vi "test - Access priority for nested read.vi"(8 "error in (no error)":errorcluster, 11 "TestCase in":refnum<class "csm-ini-variable-addon.lvclass">) -> (0 "error out":errorcluster, 3 "TestCase out":refnum<class "csm-ini-variable-addon.lvclass">)   [LabVIEW 2017, in "csm-ini-variable-addon.lvclass"]
uses:
  csm-ini-variable-addon.lvclass
  51eeedc8-b31c-488c-8392-a86325f3fef9.vi
  d661d301-294d-4a40-9fe1-44519e1c8482.vi
  51eeedc8-b31c-488c-8392-a86325f3fef9.vi/de56416b-c5bf-46ee-94c0-236aa6ebb74d.vi
  d661d301-294d-4a40-9fe1-44519e1c8482.vi/5993f3dd-cba9-41f8-9723-db1d94748cc5.vi
  INI-Static-Variable-Support/_Support/global-csm-ini-db-change-flag.vi
  <vilib>/Utility/Data Type/Get Type Information.vi
  <userlib>/_NEVSTOP/Communicable State Machine(CSM)/addons/API-String-Arugments-Support/_Support/Data To SingleElementsArray_csm.vi
  INI-Static-Variable-Support/_Support/Parse Used Session and Name.vi
  <userlib>/_NEVSTOP/Communicable State Machine(CSM)/addons/API-String-Arugments-Support/_Support/Data To API String Arguments.vi
  INI-Static-Variable-Support/_Support/INI-FGV.vi
  INI-Static-Variable-Support/_Support/Populate String with INI Variable.vi
  <userlib>/_NEVSTOP/Communicable State Machine(CSM)/addons/API-String-Arugments-Support/_Support/Convert API String Arguments to Data(variant).vi
  <userlib>/_NEVSTOP/Communicable State Machine(CSM)/addons/API-String-Arugments-Support/_Support/SingleElementsArray To Data_csm.vi
  INI-Static-Variable-Support/INI-Static-Variable-Support.lvlib
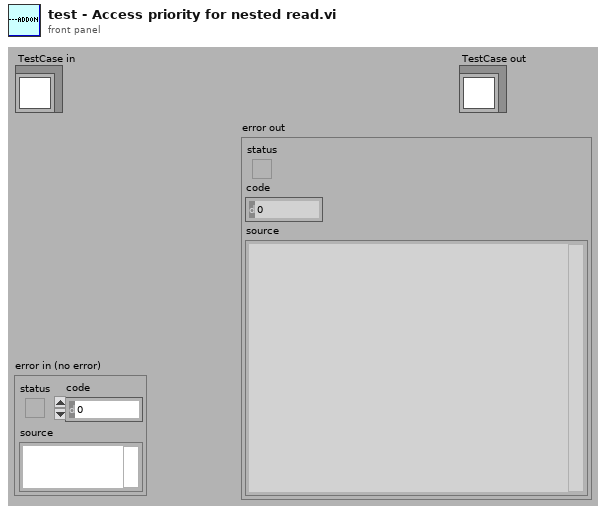
[diagram p1: front panel]
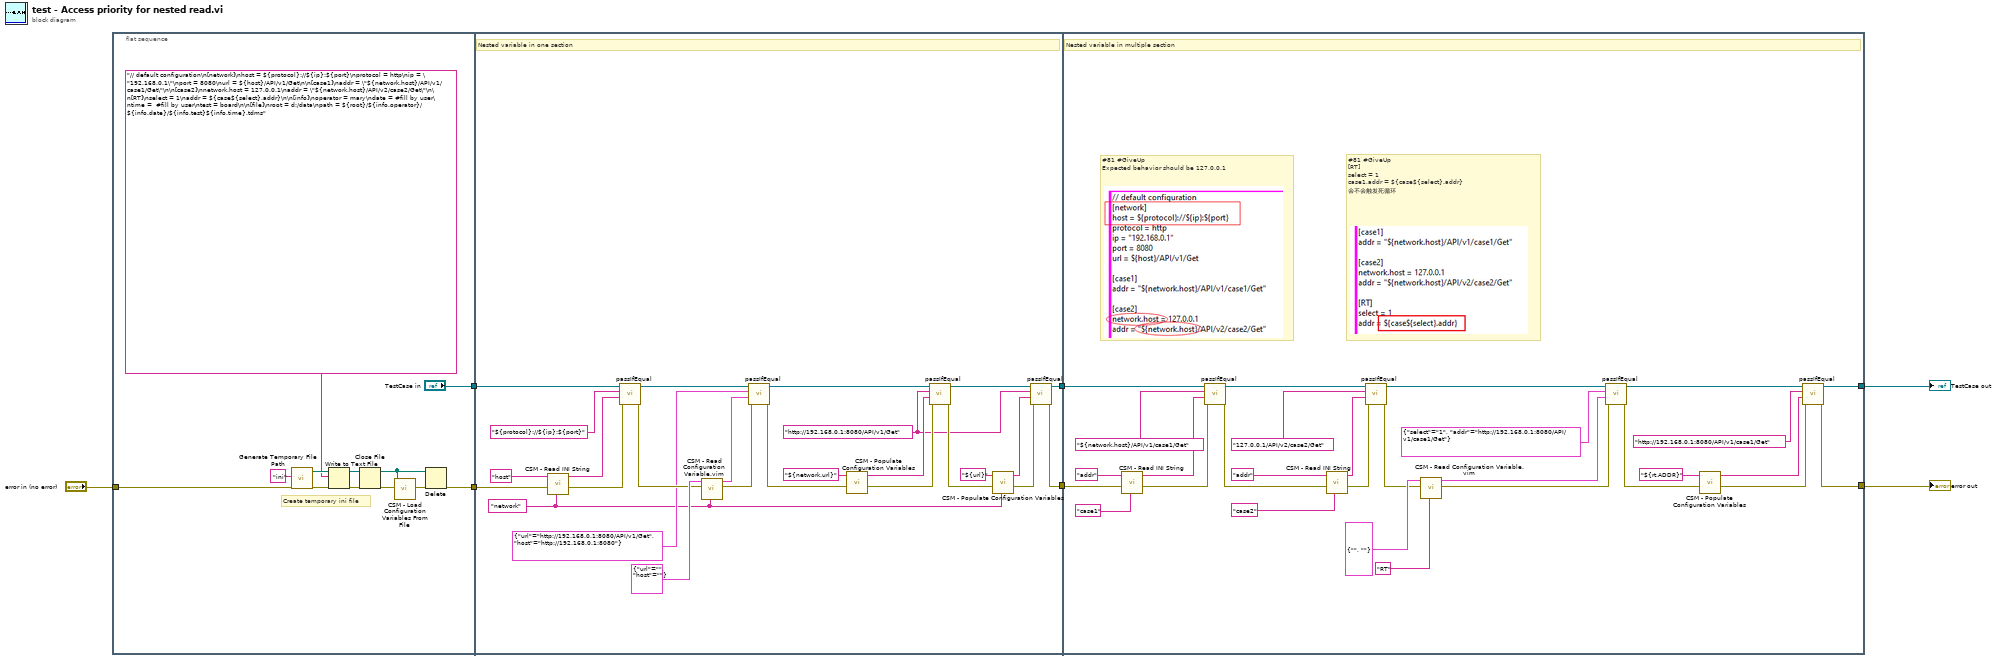
[diagram p0: block diagram]
diagram:
  n1 = flat-sequence {
    tunnel: "error in (no error)" -> [w10]
    tunnel: [w9] -> w6
    tunnel: ["TestCase in"] -> w5
    tunnel: w6 -> [w44]
    tunnel: w5 -> [w43]
    tunnel: [w21] -> w4
    tunnel: [w20] -> w3
    tunnel: w4 -> [w70]
    tunnel: w3 -> [w69]
    tunnel: [w47] -> w2
    tunnel: [w46] -> w1
    frame #0 {
      # "Create temporary ini file"
      n2 = call <vilib>:"Generate Temporary File Path.vi"("error in (no error)"=w10, "Temporary File Extension (tmp)"="ini") -> ("error out"=w19:errorcluster, "Unique Temporary File Path"=w16:path)  [unwired: 8 in]
      n3 = Write to Text File(file (use dialog)=w16, text="// default configuration\n[network]\nhost = ${protocol}://${ip}:${port}\nprotocol = http\nip = \"192.168.0.1\"\nport = 8080\nurl = ${host}/API/v1/Get\n\n[case1]\naddr = \"${network.host}/API/v1/case1/Get\"\n\n[case2]\nnetwork.host = 127.0.0.1\naddr = \"${network.host}/API/v2/case2/Get\"\n\n[RT]\nselect = 1\naddr = ${case${select}.addr}\n\n[info]\noperator = mary\ndate = #fill by user\ntime =  #fill by user\ntest = board\n\n[file]\nroot = d:/data\npath = ${root}/${info.operator}/${info.date}/${info.test}${info.time}.tdms", error in=w19) -> (refnum out=w15:refnum<file>, error out=w17:errorcluster)  [unwired: 1 in, 1 out]
      n4 = Close File(refnum=w15, error in=w17) -> (path=w11:path, error out=w14:errorcluster)
      n5 = call "CSM - Load Configuration Variables From File.vi"("error in (no error)"=w14, "Path"=w11) -> ("error out"=w12:errorcluster)  [unwired: 7 in]
      n6 = Delete(path (use dialog)=w11, error in=w12) -> (error out=w9:errorcluster)  [unwired: 3 in, 2 out]
    }
    frame #1 {
      w23 = "http://192.168.0.1:8080/API/v1/Get" ("${network.url}")
      w26 = "network" ("Section Name(\"\" as Default)")
      # "Nested variable in one section"
      n7 = call "CSM - Read INI String.vi"("Section Name(\"\" as Default)"=w26, "error in (no error)"=w44, "String in"="host") -> ("error out"=w41:errorcluster, "String out"=w42:string)  [unwired: 4 in, 1 out]
      n8 = call-dynamic "passIfEqual.vi"("error in (no error)"=w41, "y"=w42, "x"="${protocol}://${ip}:${port}" ("String in"), "TestCase in"=w43) -> ("error out"=w38:errorcluster, "TestCase out"=w36:refnum<class "csm-ini-variable-addon.lvclass">)  [unwired: 6 in]
      n9 = call "CSM - Read Configuration Variable.vim"("Section Name(\"\" as Default)"=w26, "error in (no error)"=w38, "config prototype(Cluster Prefered)"=cluster{"url":string, "host":string} {"url"="", "host"=""}) -> ("error out"=w37:errorcluster, "config out"=w35:cluster{"url":string, "host":string})  [unwired: 5 in]
      n10 = call-dynamic "passIfEqual.vi"("error in (no error)"=w37, "y"=w35, "x"=cluster{"url":string, "host":string} {"url"="http://192.168.0.1:8080/API/v1/Get", "host"="http://192.168.0.1:8080"} ("network.cluster"), "TestCase in"=w36) -> ("error out"=w31:errorcluster, "TestCase out"=w30:refnum<class "csm-ini-variable-addon.lvclass">)  [unwired: 6 in]
      n11 = call "CSM - Populate Configuration Variables.vi"("error in (no error)"=w31, "String in"="${network.url}") -> ("error out"=w28:errorcluster, "String out"=w29:string)  [unwired: 6 in]
      n12 = call-dynamic "passIfEqual.vi"("error in (no error)"=w28, "y"=w29, "x"=w23, "TestCase in"=w30) -> ("error out"=w27:errorcluster, "TestCase out"=w25:refnum<class "csm-ini-variable-addon.lvclass">)  [unwired: 6 in]
      n13 = call "CSM - Populate Configuration Variables.vi"("Section Name(\"\" as Default)"=w26, "error in (no error)"=w27, "String in"="${url}") -> ("error out"=w24:errorcluster, "String out"=w22:string)  [unwired: 5 in]
      n14 = call-dynamic "passIfEqual.vi"("error in (no error)"=w24, "y"=w22, "x"=w23, "TestCase in"=w25) -> ("error out"=w21:errorcluster, "TestCase out"=w20:refnum<class "csm-ini-variable-addon.lvclass">)  [unwired: 6 in]
    }
    frame #2 {
      # "#81 #GiveUp\nExpected behavior should be 127.0.0.1"
      # "Nested variable in multiple section"
      # "#81 #GiveUp\n[RT]\nselect = 1\ncase1.addr = ${case${select}.addr}\n会不会触发死循环"
      n15 = call "CSM - Read INI String.vi"("Section Name(\"\" as Default)"="case1" ("Section Name(\"\" as Default)"), "error in (no error)"=w70, "String in"="addr") -> ("error out"=w67:errorcluster, "String out"=w66:string)  [unwired: 4 in, 1 out]
      n16 = call-dynamic "passIfEqual.vi"("error in (no error)"=w67, "y"=w66, "x"="${network.host}/API/v1/case1/Get" ("case1.addr"), "TestCase in"=w69) -> ("error out"=w68:errorcluster, "TestCase out"=w65:refnum<class "csm-ini-variable-addon.lvclass">)  [unwired: 6 in]
      n17 = call "CSM - Read INI String.vi"("Section Name(\"\" as Default)"="case2" ("Section Name(\"\" as Default)"), "error in (no error)"=w68, "String in"="addr") -> ("error out"=w64:errorcluster, "String out"=w63:string)  [unwired: 4 in, 1 out]
      n18 = call-dynamic "passIfEqual.vi"("error in (no error)"=w64, "y"=w63, "x"="127.0.0.1/API/v2/case2/Get" ("case2.addr"), "TestCase in"=w65) -> ("error out"=w58:errorcluster, "TestCase out"=w57:refnum<class "csm-ini-variable-addon.lvclass">)  [unwired: 6 in]
      n19 = call "CSM - Read Configuration Variable.vim"("Section Name(\"\" as Default)"="RT" ("Section Name(\"\" as Default)"), "error in (no error)"=w58, "config prototype(Cluster Prefered)"=cluster{"select":string, "addr":string} {"select"="", "addr"=""}) -> ("error out"=w56:errorcluster, "config out"=w55:cluster{"select":string, "addr":string})  [unwired: 5 in]
      n20 = call-dynamic "passIfEqual.vi"("error in (no error)"=w56, "y"=w55, "x"=cluster{"select":string, "addr":string} {"select"="1", "addr"="http://192.168.0.1:8080/API/v1/case1/Get"} ("rt.cluster"), "TestCase in"=w57) -> ("error out"=w52:errorcluster, "TestCase out"=w51:refnum<class "csm-ini-variable-addon.lvclass">)  [unwired: 6 in]
      n21 = call "CSM - Populate Configuration Variables.vi"("error in (no error)"=w52, "String in"="${rt.ADDR}") -> ("error out"=w50:errorcluster, "String out"=w48:string)  [unwired: 6 in]
      n22 = call-dynamic "passIfEqual.vi"("error in (no error)"=w50, "y"=w48, "x"="http://192.168.0.1:8080/API/v1/case1/Get" ("${rt.addr}"), "TestCase in"=w51) -> ("error out"=w47:errorcluster, "TestCase out"=w46:refnum<class "csm-ini-variable-addon.lvclass">)  [unwired: 6 in]
    }
  }
  "error out" <- w2
  "TestCase out" <- w1
